vi "Refresh Configuration Parameters.vi"(6 "In Initialize?":bool, 8 "error in (no error)":errorcluster, 10 "This":T1 format="%x", 11 "Node in":refnum<class "BLS Chiller Template.lvclass"> caption="Timed Node in") -> (0 "error out":errorcluster, 2 "This out":T1 format="%x", 3 "Node out":refnum<class "BLS Chiller Template.lvclass"> caption="Timed Node out")   [LabVIEW 2023, in "BLS Chiller Template.lvlib" / "BLS Chiller Template.lvclass"]
uses:
  BLS Chiller Template.lvclass
  Program Files/National Instruments/ADAS Replay HIL/EVO SDK/Linux RT/evoLabVIEWAPI/evoPluginSDK.lvlibp/VIs/TypeDefs/Handle.ctl
  Configuration Params.ctl
  <vilib>/ADAS Replay HIL/Template Node/Plugin/Template Node/Common Configuration Params.ctl
  BLS Chiller Template.lvclass/BLS Chiller Template.ctl
  <vilib>/ADAS Replay HIL/Template Node/Plugin/Template Node/Template Node.lvclass/Template Node.ctl
  c3f9980b-0202-4a5c-a15f-679fa66f24a8.vi
  <vilib>/Utility/error.llb/Trim Whitespace One-Sided.vi
  <vilib>/ADAS Replay HIL/AdasCommonUtilities/Config/Data Converter/SubVIs/Replace JSON SubArray with String.vi
  <vilib>/ADAS Replay HIL/AdasCommonUtilities/Config/Data Converter/SubVIs/Variant From Data Node.vi
  <vilib>/ADAS Replay HIL/Template Node/Plugin/Template Node/Write Common Config Params.vi
  Program Files/National Instruments/ADAS Replay HIL/EVO SDK/Linux RT/evoLabVIEWAPI/evoPluginSDK.lvlibp
  <vilib>/ADAS Replay HIL/Template Node/Plugin/Template Node/Template Node.lvclass
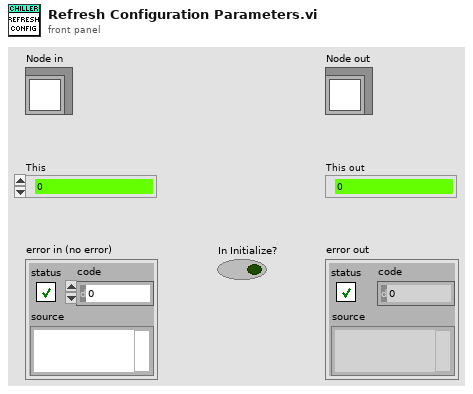
[diagram p1: front panel]
types:
  T1 = typedef "evoPluginSDK.lvlibp/Handle.ctl" = u64
  T2 = typedef "BLS Chiller Template.lvlib/BLS Chiller Template.lvclass/Configuration Params.ctl" = cluster{"Common":T3}
  T3 = typedef "Template Node.lvlib/Template Node.lvclass/Common Configuration Params.ctl" = cluster{"Iteration Interval (s)":dbl, "T0 (ns)":u64, "Priority":i32, "Processor":i32, "Wait in Ready State":bool}
  T4 = cluster{"Config JSON":string, "Plugin Name":string, "Instance ID":string}
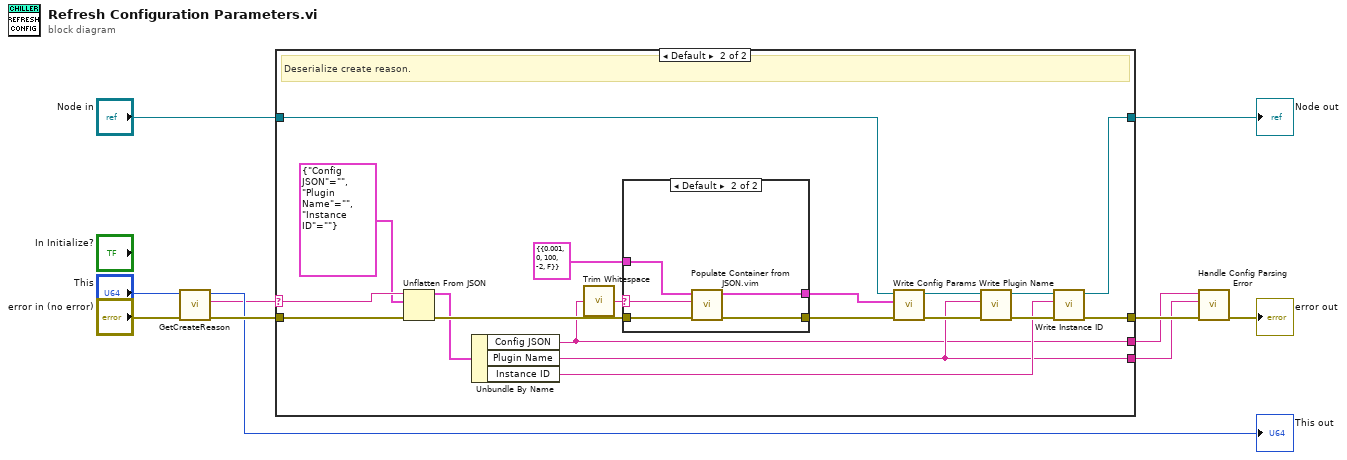
[diagram p0: block diagram]
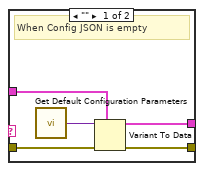
[diagram p3: hidden frame]
diagram:
  n1 = call "GetCreateReason.vi"("error in (no error)"="error in (no error)", "This"="This") -> ("error out"=w7:errorcluster, "Create Reason"=w5:string, "This"=→"This out":T1)  [unwired: 7 in]
  n2 = case shown="Default" w5 {
    selector: w5 -> [_ w26]
    tunnel: w7 -> [w12 w32]
    tunnel: [w12 w21] -> w3
    tunnel: "Node in" -> [w13 w28]
    tunnel: [w13 w19] -> w8
    tunnel: [_ w17] -> w2
    tunnel: [_ w16] -> w1
    frame "" {
      # "If no CreateReason was provided, this is likely because it hasn't been implemented in the execution code, and configuration parameters will not be settable. Leaving this here for early development to avoid difficult-to-debug issues. Will want to reconsider how this is handled moving forward."
    }
    frame Default {
      # "Deserialize create reason."
      n3 = Unflatten From JSON(JSON string=w26, type and defaults=T4 {"Config JSON"="", "Plugin Name"="", "Instance ID"=""}, error in (no error)=w32) -> (value=w24:T4, error out=w27:errorcluster)  [unwired: 4 in]
      n4 = Unbundle By Name(w24) -> ("Config JSON"=w16:string, "Plugin Name"=w17:string, "Instance ID"=w18:string)
      n5 = call <vilib>:"Trim Whitespace.vi"("string"=w16) -> ("trimmed string"=w14:string)  [unwired: 1 in]
      n6 = case shown="Default" w14 {
        selector: w14 -> [_ w38]
        tunnel: [w36 w42] -> w31
        tunnel: [w33 w41] -> w29
        tunnel: w27 -> [w37 w40]
        tunnel: T2 {"Common"={"Iteration Interval (s)"=0.001, "T0 (ns)"=0, "Priority"=100, "Processor"=-2, "Wait in Ready State"=FALSE}} ("Default Parameters") -> [w34 w39]
        frame "" {
          # "When Config JSON is empty"
          n7 = call "Get Default Configuration Parameters.vi"() -> ("Default Config Params"=w35:variant)
          n8 = Variant To Data(error in=w37, type=w34, Variant=w35) -> (data=w33:T2, error out=w36:errorcluster)
        }
        frame Default {
          n9 = call "Populate Container from JSON.vim"("error in (no error)"=w40, "JSON string In"=w38, "Container In"=w39) -> ("error out"=w42:errorcluster, "Container Out"=w41:T2)  [unwired: 6 in, 1 out]
        }
      }
      n10 = call "Write Config Params.vi"("error in"=w31, "Default Parameters"=w29, "Node in"=w28) -> ("error out"=w30:errorcluster, "Node out"=w22:refnum<class "BLS Chiller Template.lvclass">)  [unwired: 7 in]
      n11 = call <vilib>:"Write Plugin Name.vi"("error in"=w30, "Plugin Name"=w17, "Template Node in"=w22) -> ("error out"=w23:errorcluster, "Template Node out"=w20:refnum<class "BLS Chiller Template.lvclass">)  [unwired: 7 in]
      n12 = call <vilib>:"Write Instance ID.vi"("error in"=w23, "Instance ID"=w18, "Template Node in"=w20) -> ("error out"=w21:errorcluster, "Template Node out"=w19:refnum<class "BLS Chiller Template.lvclass">)  [unwired: 7 in]
    }
  }
  "Node out" <- w8
  n13 = call <vilib>:"Handle Config Parsing Error.vi"("error in"=w3, "Plugin Name"=w2, "Config JSON"=w1) -> ("error out"=→"error out":errorcluster)  [unwired: 8 in]
